vi "crete socket.vi"(8 "error in (no error)":errorcluster, 11 "Socket in":refnum<class "Socket.lvclass">) -> (0 "error out":errorcluster, 3 "Socket out":refnum<class "Socket.lvclass">)   [LabVIEW 2018, in "Socket.lvclass"]
uses:
  Socket.lvclass
  Socket.lvclass/Socket.ctl
  <vilib>/addons/zeromq/zmq_context.lvclass
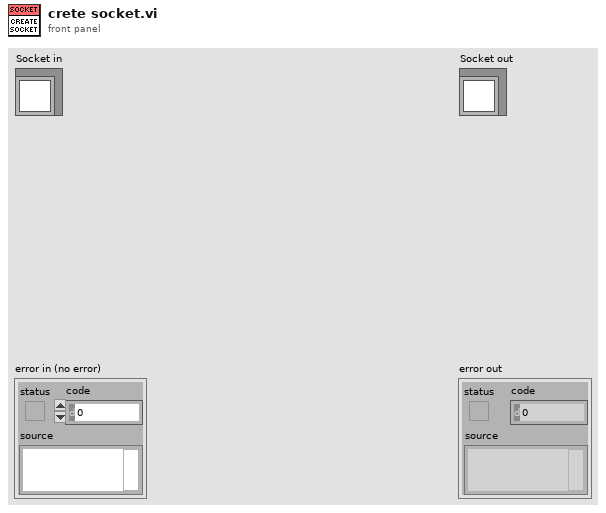
[diagram p1: front panel]
types:
  T1 = typedef "zeromq.lvlib/socket_type.ctl" = enum8{"ZMQ_PAIR", "ZMQ_PUB", "ZMQ_SUB", "ZMQ_REQ", "ZMQ_REP", "ZMQ_DEALER", "ZMQ_ROUTER", "ZMQ_PULL", "ZMQ_PUSH", "ZMQ_XPUB", "ZMQ_XSUB", "ZMQ_STREAM", "ZMQ_SERVER", "ZMQ_CLIENT", "ZMQ_RADIO", "ZMQ_DISH", "ZMQ_GATHER", "ZMQ_SCATTER", "ZMQ_DGRAM"}
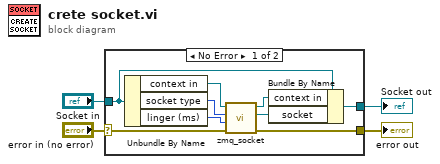
[diagram p0: block diagram]
diagram:
  n1 = case shown="No Error" "error in (no error)" {
    selector: "error in (no error)" -> [w13 w15]
    tunnel: [w12 w15] -> w3
    tunnel: [w9 w14] -> w1
    tunnel: "Socket in" -> [w10 w14]
    frame No Error {
      n2 = Unbundle By Name(w10) -> ("context in"=w11:refnum<class "zmq_context.lvclass">, "socket type"=w6:T1, "linger (ms)"=w5:i32)
      n3 = call <vilib>:"zmq_socket.vi"("error in"=w13, "linger (ms)"=w5, "socket type"=w6, "context in"=w11) -> ("error out"=w12:errorcluster, "socket out"=w7:refnum<class "zmq_socket.lvclass">, "context out"=w8:refnum<class "zmq_context.lvclass">)  [unwired: 1 in]
      n4 = Bundle By Name(cluster=w10, "context in"=w8, "socket"=w7) -> (w9:refnum<class "Socket.lvclass">)
    }
    frame Error {
    }
  }
  "error out" <- w3
  "Socket out" <- w1
